vi "test_libssh2_session_callback_set - no handler.vi"() -> ()   [LabVIEW 2017, in "integration_tests.lvlib"]
uses:
  integration_tests.lvlib
  libssh2/libssh2_session_callback_type.ctl
  libssh2/libssh2_session_handshake_tcp.vi
  libssh2/libssh2_init_default.vi
  <vilib>/Utility/tcp.llb/TCP Get Raw Net Object.vi
  libssh2/libssh2_session_handshake_socket.vi
  libssh2/libssh2.lvlib
  support/support.lvlib
  <vilib>/PNR/Transparent Assertions/Transparent Assertions/Transparent Assertions.lvlib
panel:
  out "error out":errorcluster
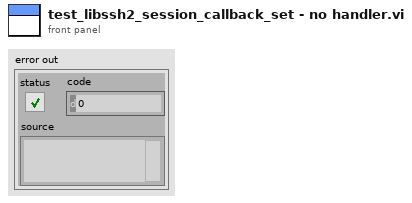
[diagram p1: front panel]
types:
  T1 = typedef "libssh2.lvlib/libssh2_session_callback_type.ctl" = enum16{"Ignore", "Debug", "Disconnect", "MAC Error", "X11", "Send", "Receive", "Auth Agent", "Auth Agent Identities", "Auth Agent Sign"}
  T2 = typedef "libssh2.lvlib/Session Refnum.ctl" = refnum<k1>
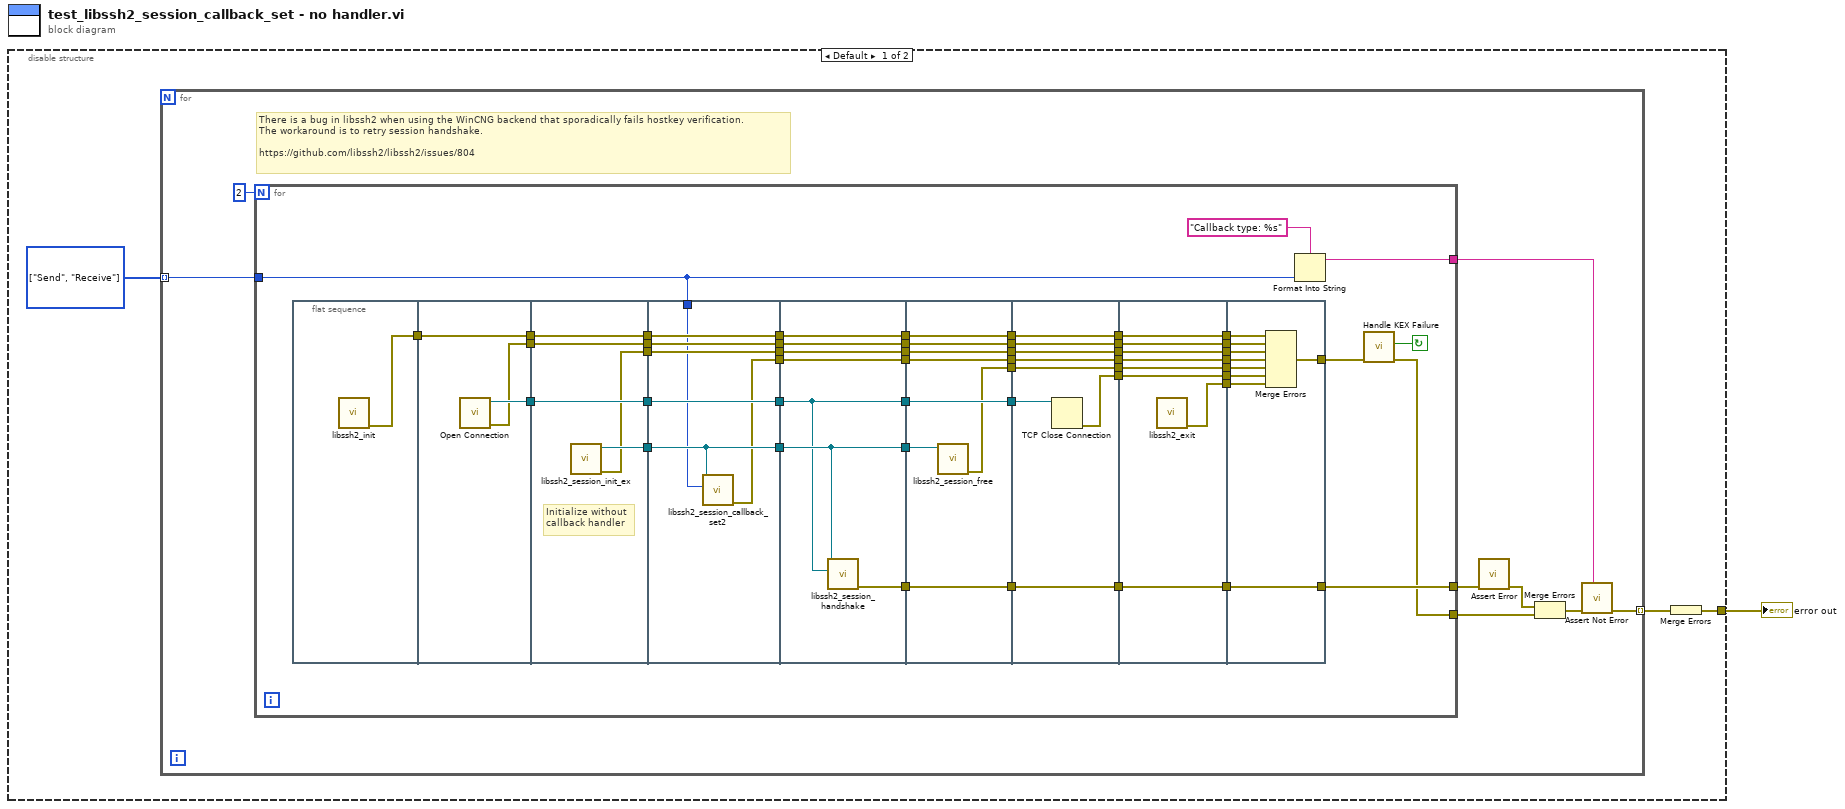
[diagram p0: block diagram]
diagram:
  n1 = disable-structure shown="Default" {
    disable-tunnel: [w2 _] -> w1
    frame condition #0 (active) {
      w3 = T1[] [enum."Send", enum."Receive"] items=["Ignore", "Debug", "Disconnect", "MAC Error", "X11", "Send", "Receive", "Auth Agent", "Auth Agent Identities", "Auth Agent Sign"]
      n2 = for {
        tunnel: [w10] -> w4 mode=indexing
        tunnel: w3 -> [w12] mode=indexing
        # "There is a bug in libssh2 when using the WinCNG backend that sporadically fails hostkey verification.\nThe workaround is to retry session handshake.\n\nhttps://github.com/libssh2/libssh2/issues/804"
        n3 = for {
          N: 2 -> [_]
          tunnel: w12 -> [w19]
          tunnel: [w17] -> w11
          tunnel: [w16] -> w7
          tunnel: [w13] -> w9
          stop <- w14 continue-if-true
          n4 = flat-sequence {
            tunnel: [w64] -> w63
            tunnel: [w67] -> w62
            tunnel: w63 -> [w66]
            tunnel: [w66] -> w61
            tunnel: [w65] -> w60
            tunnel: w62 -> [w72]
            tunnel: [w72] -> w59
            tunnel: w61 -> [w71]
            tunnel: [w71] -> w58
            tunnel: w60 -> [w70]
            tunnel: [w70] -> w57
            tunnel: [w69] -> w56
            tunnel: [w68] -> w55
            tunnel: w59 -> [w79]
            tunnel: [w79] -> w54
            tunnel: w58 -> [w78]
            tunnel: [w78] -> w53
            tunnel: w57 -> [w77]
            tunnel: [w77] -> w52
            tunnel: w56 -> [w75]
            tunnel: [w75] -> w51
            tunnel: w55 -> [w76]
            tunnel: [w76] -> w50
            tunnel: [w74] -> w49
            tunnel: w19 -> [w73]
            tunnel: w54 -> [w82]
            tunnel: [w82] -> w48
            tunnel: w53 -> [w86]
            tunnel: [w86] -> w47
            tunnel: w52 -> [w85]
            tunnel: [w85] -> w46
            tunnel: [w84] -> w43
            tunnel: w51 -> [w84]
            tunnel: w50 -> [w83]
            tunnel: [w83] -> w45
            tunnel: w49 -> [w81]
            tunnel: [w81] -> w44
            tunnel: [w80] -> w42
            tunnel: w48 -> [w94]
            tunnel: [w94] -> w41
            tunnel: w47 -> [w93]
            tunnel: [w93] -> w40
            tunnel: w46 -> [w92]
            tunnel: [w92] -> w39
            tunnel: w45 -> [w91]
            tunnel: [w91] -> w38
            tunnel: w44 -> [w90]
            tunnel: [w90] -> w37
            tunnel: w43 -> [w89]
            tunnel: [w88] -> w36
            tunnel: [w87] -> w35
            tunnel: w42 -> [w87]
            tunnel: w41 -> [w102]
            tunnel: w40 -> [w101]
            tunnel: [w101] -> w34
            tunnel: w39 -> [w100]
            tunnel: [w100] -> w33
            tunnel: [w99] -> w32
            tunnel: w38 -> [w98]
            tunnel: [w98] -> w31
            tunnel: w37 -> [w97]
            tunnel: [w97] -> w30
            tunnel: [w96] -> w29
            tunnel: w36 -> [w96]
            tunnel: [w95] -> w28
            tunnel: w35 -> [w95]
            tunnel: w34 -> [w110]
            tunnel: [w110] -> w27
            tunnel: w33 -> [w109]
            tunnel: [w109] -> w26
            tunnel: w32 -> [w108]
            tunnel: [w108] -> w25
            tunnel: [w107] -> w24
            tunnel: w31 -> [w106]
            tunnel: [w106] -> w23
            tunnel: w30 -> [w105]
            tunnel: [w105] -> w22
            tunnel: [w104] -> w21
            tunnel: w29 -> [w104]
            tunnel: [w103] -> w20
            tunnel: w28 -> [w103]
            tunnel: w27 -> [w119]
            tunnel: w26 -> [w118]
            tunnel: w25 -> [w117]
            tunnel: w24 -> [w116]
            tunnel: w23 -> [w115]
            tunnel: w22 -> [w114]
            tunnel: w21 -> [w113]
            tunnel: w20 -> [w112]
            tunnel: [w112] -> w16
            tunnel: [w111] -> w15
            frame #0 {
              n5 = call-poly "libssh2_init.vi"() -> ("error out"=w64:errorcluster)  [unwired: 11 in]
            }
            frame #1 {
              n6 = call "Open Connection.vi"() -> ("error out"=w65:errorcluster, "connection ID"=w67:refnum<k5>)  [unwired: 10 in]
            }
            frame #2 {
              # "Initialize without\ncallback handler"
              n7 = call "libssh2_session_init_ex.vi"() -> ("error out"=w68:errorcluster, "session"=w69:T2)  [unwired: 10 in]
            }
            frame #3 {
              n8 = call "libssh2_session_callback_set2.vi"("callback type"=w73, "session"=w75) -> ("error out"=w74:errorcluster)  [unwired: 8 in, 1 out]
            }
            frame #4 {
              n9 = call-poly "libssh2_session_handshake.vi"("tcp connection"=w82, "session"=w84) -> ("error out"=w80:errorcluster)  [unwired: 9 in]
            }
            frame #5 {
              n10 = call "libssh2_session_free.vi"("session"=w89) -> ("error out"=w88:errorcluster)  [unwired: 10 in]
            }
            frame #6 {
              n11 = TCP Close Connection(connection ID=w102) -> (error out=w99:errorcluster)  [unwired: 2 in, 1 out]
            }
            frame #7 {
              n12 = call "libssh2_exit.vi"() -> ("error out"=w107:errorcluster)  [unwired: 11 in]
            }
            frame #8 {
              n13 = Merge Errors(w119, w118, w115, w114, w113, w117, w116) -> (w111:errorcluster)
            }
          }
          n14 = Format Into String(format string="Callback type: %s", w19) -> (resulting string=w17:string)  [unwired: 2 in, 1 out]
          n15 = call "Handle KEX Failure.vi"("error in (no error)"=w15) -> ("error out"=w13:errorcluster, "KEX Failure"=w14:bool)  [unwired: 9 in]
        }
        n16 = call <vilib>:"Assert Error.vi"("error in (no error)"=w7) -> ("error out"=w5:errorcluster)  [unwired: 10 in]
        n17 = Merge Errors(w5, w9) -> (w6:errorcluster)
        n18 = call <vilib>:"Assert Not Error.vi"("Message (\"\")"=w11, "error in (no error)"=w6) -> ("error out"=w10:errorcluster)  [unwired: 9 in]
      }
      n19 = Merge Errors(w4) -> (w2:errorcluster)
    }
    frame condition #1 {
    }
  }
  "error out" <- w1
